vi "Teardown.vi"(8 "error in (no error)":errorcluster, 11 "LUnit Configuration Manager Test In":refnum<class "Configuration Manager Test.lvclass">) -> (0 "error out":errorcluster, 3 "LUnit Configuration Manager Test Out":refnum<class "Configuration Manager Test.lvclass">)   [LabVIEW 2020, in "Configuration Manager Test.lvclass"]
uses:
  Configuration Manager Test.lvclass
  Configuration Manager Test.lvclass/Configuration Manager Test.ctl
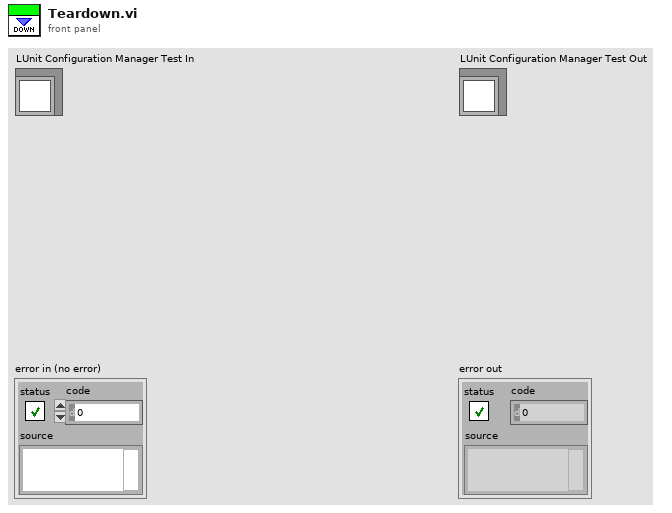
[diagram p1: front panel]
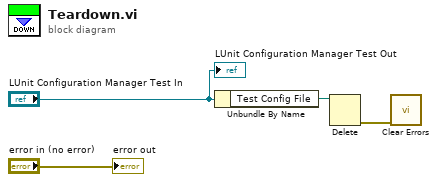
[diagram p0: block diagram]
diagram:
  n1 = Unbundle By Name("LUnit Configuration Manager Test In") -> ("Test Config File"=w2:path)
  n2 = Delete(path (use dialog)=w2) -> (error out=w1:errorcluster)  [unwired: 4 in, 2 out]
  n3 = call <vilib>:"Clear Errors.vi"("error in (no error)"=w1) -> ()  [unwired: 5 in, 2 out]
  "error out" <- "error in (no error)"
  "LUnit Configuration Manager Test Out" <- "LUnit Configuration Manager Test In"
